vi "Swerve Drive Drive.vi"(6 "Speed Multiplier":dbl, 7 "Description":string, 8 "Command Info In":T1, 9 "Face Joystick Axes":cluster{"X":dbl, "Y":dbl}, 10 "Strafe Joystick Axes":cluster{"X":dbl, "Y":dbl}, 11 "Trigger Axes":cluster{"Left":dbl, "Right":dbl}) -> (0 "Command Info Out":T1)   [LabVIEW 2015]
uses:
  <vilib>/Rock Robotics/WPI/Framework/Command Status Info.ctl
  <vilib>/Rock Robotics/WPI/Framework/Completion Status.ctl
  <vilib>/Rock Robotics/WPI/Framework/Completion Notifier.ctl
  Implementation/Swerve Drive Operations.ctl
  Implementation/Swerve Drive Setpoints.ctl
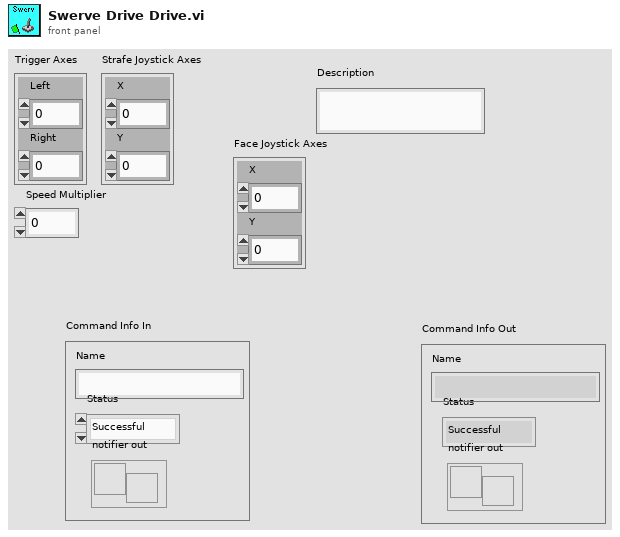
[diagram p1: front panel]
types:
  T1 = typedef "Command Status Info.ctl" = cluster{"Name":string, "Status":T2, "notifier out":T3}
  T2 = typedef "Completion Status.ctl" = enum16{"Successful", "Aborted", "Incomplete"}
  T3 = typedef "Completion Notifier.ctl" = refnum<notifier>
  T4 = typedef "Swerve Drive Setpoints.ctl" = cluster{"Operation":T5, "Duration":dbl, "Joystick":cluster{"Trigger Axes":cluster{"Left":dbl, "Right":dbl}, "Strafe Joystick Axes":cluster{"X":dbl, "Y":dbl}, "Face Joystick Axes":cluster{"X":dbl, "Y":dbl}}, "Position":cluster{"X":dbl, "Y":dbl, "R":dbl}, "Speed Multiplier":dbl}
  T5 = typedef "Swerve Drive Operations.ctl" = enum16{"Reserve", "Read Current", "Immeditate", "Drive", "Go to Coordinates"}
  T6 = cluster{"Trigger Axes":cluster{"Left":dbl, "Right":dbl}, "Strafe Joystick Axes":cluster{"X":dbl, "Y":dbl}, "Face Joystick Axes":cluster{"X":dbl, "Y":dbl}}
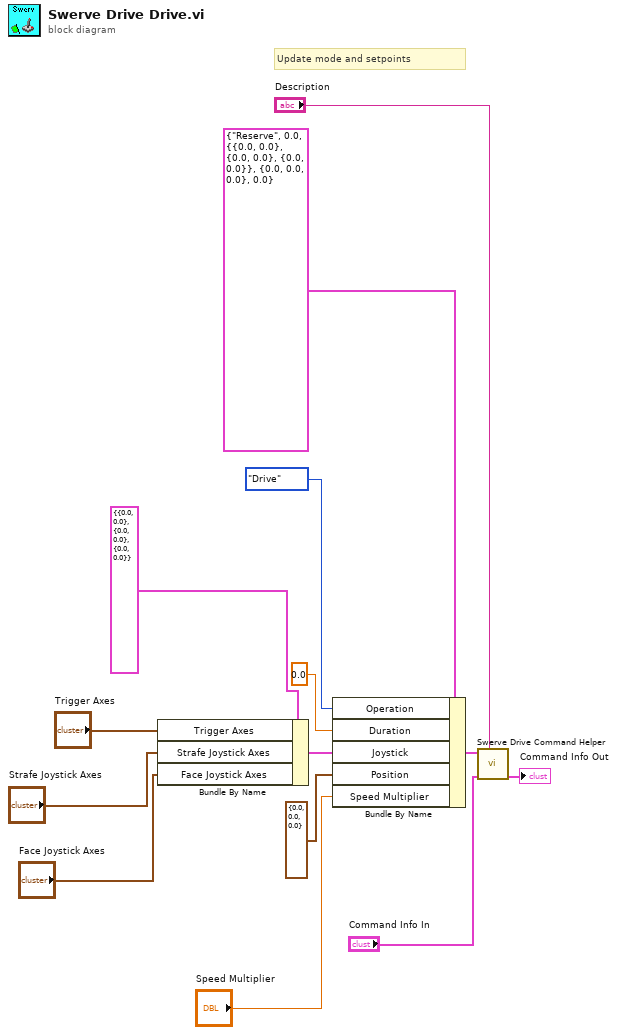
[diagram p0: block diagram]
diagram:
  # "Update mode and setpoints"
  n1 = Bundle By Name(cluster=T6 {"Trigger Axes"={"Left"=0.0, "Right"=0.0}, "Strafe Joystick Axes"={"X"=0.0, "Y"=0.0}, "Face Joystick Axes"={"X"=0.0, "Y"=0.0}} ("Joystick"), "Trigger Axes"="Trigger Axes", "Strafe Joystick Axes"="Strafe Joystick Axes", "Face Joystick Axes"="Face Joystick Axes") -> (w4:T6)
  n2 = Bundle By Name(cluster=T4 {"Operation"=enum."Reserve", "Duration"=0.0, "Joystick"={"Trigger Axes"={"Left"=0.0, "Right"=0.0}, "Strafe Joystick Axes"={"X"=0.0, "Y"=0.0}, "Face Joystick Axes"={"X"=0.0, "Y"=0.0}}, "Position"={"X"=0.0, "Y"=0.0, "R"=0.0}, "Speed Multiplier"=0.0} ("SubSystem Data"), "Operation"=Swerve_Drive_Operations."Drive", "Duration"=0.0, "Joystick"=w4, "Position"=cluster{"X":dbl, "Y":dbl, "R":dbl} {"X"=0.0, "Y"=0.0, "R"=0.0}, "Speed Multiplier"="Speed Multiplier") -> (w10:T4)
  n3 = call "Swerve Drive Command Helper.vi"("Description"="Description", "Command Info In"="Command Info In", "SubSystem Data"=w10) -> ("Command Info Out"=→"Command Info Out":T1)  [unwired: 7 in, 1 out]
